vi "Task Active--Const.vi"() -> (3 "Task Active Command":string)   [LabVIEW 2017, in "Communications Library.lvlib"]
uses:
  Communications Library.lvlib
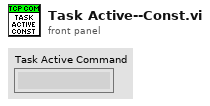
[diagram p1: front panel]
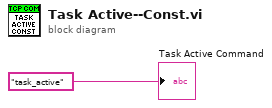
[diagram p0: block diagram]
diagram:
  "Task Active Command" <- "task_active" ("data in")
